vi "Log Error To File.vi"(8 "Error In":errorcluster, 10 "Error Level":T1=enum."System Error", 11 "Error Handler in":refnum<class "Error Handler.lvclass">) -> (0 "error out":errorcluster, 3 "Error Handler out":refnum<class "Error Handler.lvclass">)   [LabVIEW 2012, in "Architecture.lvlib" / "Error Handler.lvclass"]
uses:
  Error Handler.lvclass
  EH Action.ctl
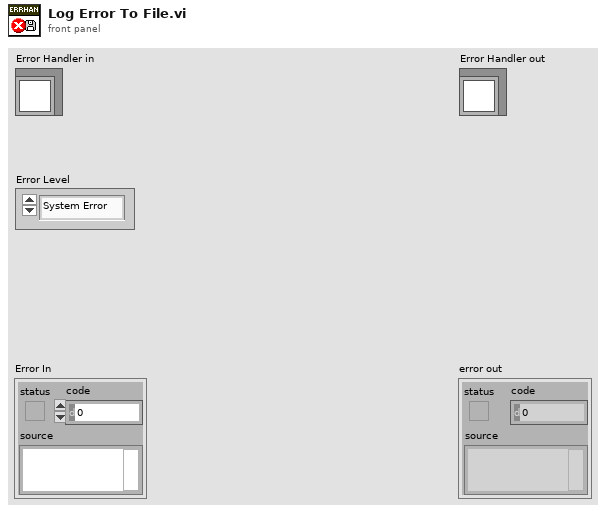
[diagram p1: front panel]
types:
  T1 = typedef "Architecture.lvlib/Error Handler.lvclass/EH Action.ctl" = enum16{"Define Threads", "Close", "System Error", "Wash Cycle Error", "Minor Error", "Initialize"}
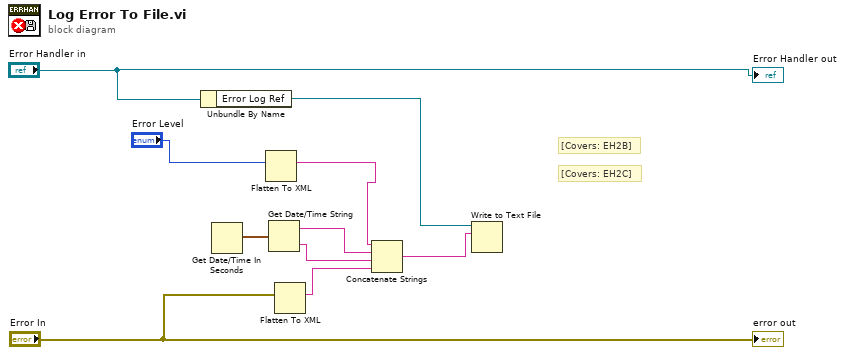
[diagram p0: block diagram]
diagram:
  # "[Covers: EH2C]"
  # "[Covers: EH2B]"
  n1 = Unbundle By Name("Error Handler in") -> ("Error Log Ref"=w9:refnum<file>)
  n2 = Get Date/Time In Seconds() -> (seconds since 1Jan1904=w6:timestamp)
  n3 = Flatten To XML(anything="Error Level") -> (xml string=w2:string)
  n4 = Get Date/Time String(seconds (now)=w6) -> (date string=w4:string, time string=w5:string)  [unwired: 2 in]
  n5 = Flatten To XML(anything="Error In") -> (xml string=w7:string)
  n6 = Concatenate Strings(w2, w4, w5, w7) -> (w1:string)
  n7 = Write to Text File(file (use dialog)=w9, text=w1) -> ()  [unwired: 2 in, 3 out]
  "error out" <- "Error In"
  "Error Handler out" <- "Error Handler in"
